vi "Build Installer.vi"(8 "error in (no error)":errorcluster, 11 "PostBuildSupport in":refnum<class "PostBuildSupport.lvclass">) -> (0 "error out":errorcluster, 3 "PostBuildSupport out":refnum<class "PostBuildSupport.lvclass">)   [LabVIEW 2019, in "PostBuildSupport.lvclass"]
uses:
  PostBuildSupport.lvclass
  PostBuildSupport.lvclass/PostBuildSupport.ctl
  <vilib>/AppBuilder/AB_API_Simple/Build (path).vi
  <vilib>/AppBuilder/AB_API_Simple/NI_App_Builder_API.lvlib
panel:
  out "Progress Bar":u8(slide) caption="Opening PPMS Monitor and Control Installer" scale=0.0..100.0
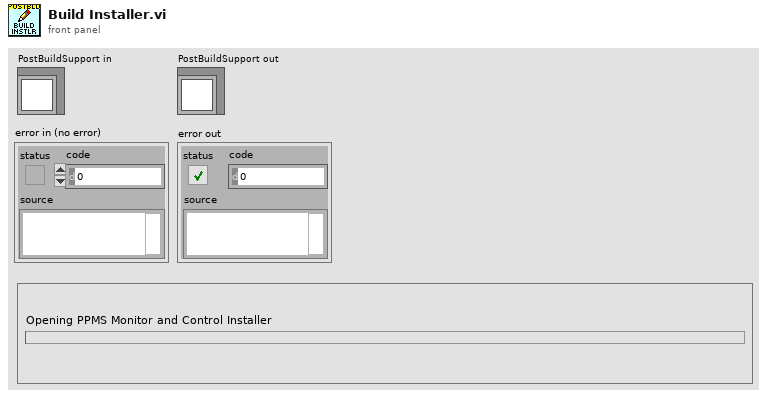
[diagram p1: front panel]
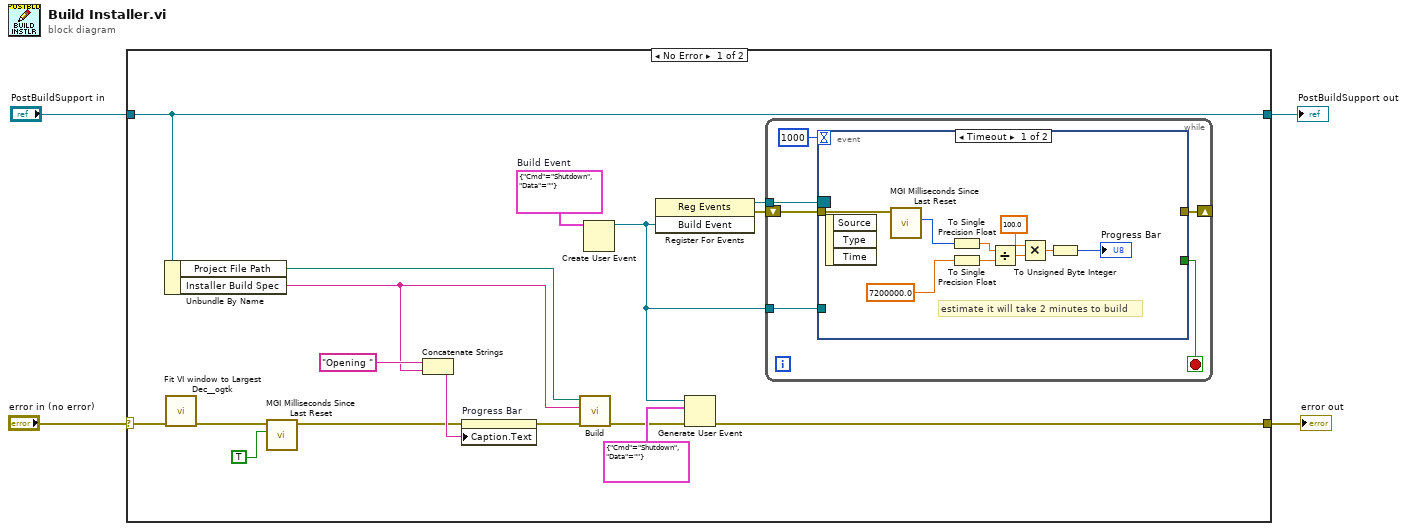
[diagram p0: block diagram]
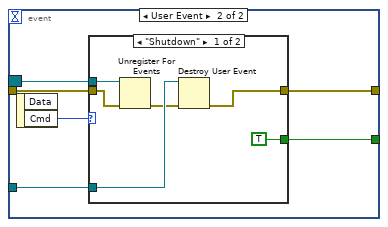
[diagram p2: hidden frame]
diagram:
  n1 = case shown="No Error" "error in (no error)" {
    selector: "error in (no error)" -> [w19 w51]
    tunnel: "PostBuildSupport in" -> [w21 w50]
    tunnel: [w10 w51] -> w2
    tunnel: [w21 w50] -> w1
    frame No Error {
      w16 = cluster{"Cmd":enum16{"Shutdown"}, "Data":string} {"Cmd"=enum."Shutdown", "Data"=""}  # Build Event
      n2 = Unbundle By Name(w21) -> ("Project File Path"=w6:path, "Installer Build Spec"=w5:string)
      n3 = call <userlib>:"Fit VI window to Largest Dec__ogtk.vi"("error in (no error)"=w19) -> ("error out"=w8:errorcluster)  [unwired: 5 in, 1 out]
      n4 = call <userlib>:"MGI Milliseconds Since Last Reset.vi"("Reset (F)"=TRUE, "Error In"=w8) -> ("Error Out"=w7:errorcluster)  [unwired: 4 in, 1 out]
      n5 = Concatenate Strings("Opening " ("string"), w5) -> (w18:string)
      n6 = property on="Progress Bar" class="Slide (strict)"(error in=w7, "Caption.Text"=w18) -> (error out=w17:errorcluster)  [unwired: 1 in, 1 out]
      n7 = call-poly <vilib>:"Build.vi"("error in (no error)"=w17, "Name of build specification (if empty: build all)"=w5, "Path to project"=w6) -> ("error out"=w14:errorcluster)  [unwired: 7 in, 1 out]
      n8 = Create User Event(user event datatype=w16) -> (user event=w12:refnum<user-event>)  [unwired: 1 in, 1 out]
      n9 = register-events(w12) -> (reference out=w13:refnum<event-registration>, error out=w11:errorcluster)  [unwired: 2 in]
      n10 = Generate User Event(user event=w12, event data cluster=cluster{"Cmd":enum16{"Shutdown"}, "Data":string} {"Cmd"=enum."Shutdown", "Data"=""} ("event data"), error in=w14) -> (error out=w10:errorcluster)  [unwired: 1 in, 1 out]
      n11 = while {
        tunnel: w13 -> [w27]
        tunnel: w12 -> [w26]
        shift-right: [w24] -> _
        shift-left: w11 -> [w25]
        stop <- w23 stop-if-true
        n12 = event shown="[0] Timeout" {
          selector: w27 -> [_ w40]
          dyn-events: _ -> [_ _]
          timeout: 1000 -> [_ _]
          tunnel: w26 -> [_ w42]
          tunnel: w25 -> [w30 w41]
          tunnel: [_ w39] -> w24
          tunnel: [_ w38] -> w23
          event Timeout {
            # "estimate it will take 2 minutes to build"
            n13 = event-data() -> ()  [unwired: 1 in, 3 out]
            n14 = call <userlib>:"MGI Milliseconds Since Last Reset.vi"("Error In"=w30) -> ("ms"=w29:u32)  [unwired: 5 in, 1 out]
            n15 = To Single Precision Float(number=w29) -> (single precision float=w33:sgl)
            n16 = To Single Precision Float(number=sgl 7200000.0) -> (single precision float=w32:sgl)
            n17 = Divide(x=w33, y=w32) -> (x/y=w34:sgl)
            n18 = Multiply(x=sgl 100.0, y=w34) -> (x*y=w36:sgl)
            n19 = To Unsigned Byte Integer(number=w36) -> (unsigned 8bit integer=→"Progress Bar":u8)
          }
          event User Event {
            n20 = event-data() -> ("Cmd"=w37:enum16{"Shutdown"})  [unwired: 1 in, 1 out]
            n21 = case shown="\"Shutdown\"" w37 {
              tunnel: [TRUE _] -> w38
              tunnel: w40 -> [w47 _]
              tunnel: [w43 w49] -> w39
              tunnel: w41 -> [w46 w49]
              tunnel: w42 -> [w45 _]
              frame "Shutdown" {
                n22 = Unregister For Events(event registration refnum=w47, error in=w46) -> (error out=w44:errorcluster)
                n23 = Destroy User Event(user event=w45, error in=w44) -> (error out=w43:errorcluster)
              }
              frame Default {
              }
            }
          }
        }
      }
    }
    frame Error {
    }
  }
  "error out" <- w2
  "PostBuildSupport out" <- w1
